vi "topicRequest_Reply_Decode.vi"(1 "Topic Request Reply":string) -> (0 "Topic Request Reply":T1)   [LabVIEW 2013]
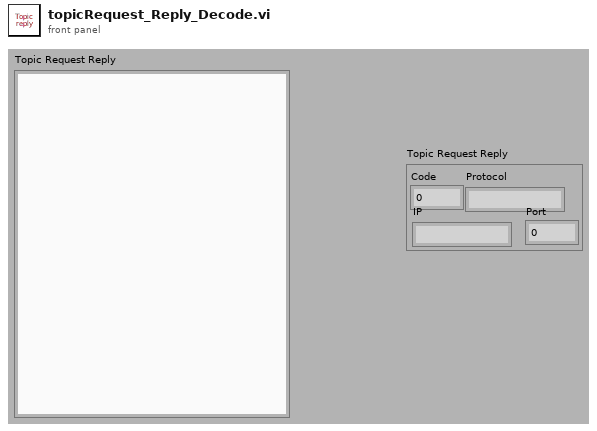
[diagram p1: front panel]
types:
  T1 = cluster{"Protocol":string, "Code":i32, "IP":string, "Port":i32}
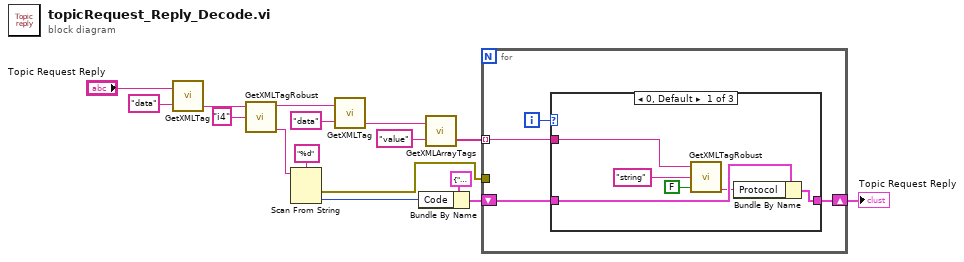
[diagram p0: block diagram]
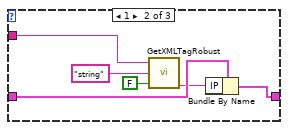
[diagram p2: hidden frame]
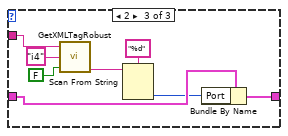
[diagram p3: hidden frame]
diagram:
  n1 = call "GetXMLTag.vi"("Tag"="data" ("ArrayTag"), "String"="Topic Request Reply") -> ("Value"=w12:string)  [unwired: 2 out]
  n2 = call "GetXMLTagRobust.vi"("Tag"="i4", "String"=w12) -> ("value"=w10:string, "String w/o Tag"=w4:string)  [unwired: 1 in, 2 out]
  n3 = Scan From String(format string="%d", input string=w10) -> (error out=w1:errorcluster, output 1=w9:i32)  [unwired: 3 in, 2 out]
  n4 = call "GetXMLTag.vi"("Tag"="data", "String"=w4) -> ("Value"=w3:string)  [unwired: 2 out]
  n5 = Bundle By Name(cluster=T1 {"Protocol"="", "Code"=0, "IP"="", "Port"=0} ("Topic Request Reply"), "Code"=w9) -> (w7:T1)
  n6 = call "GetXMLArrayTags.vi"("ArrayTag"="value", "String"=w3) -> ("Array"=w6:string[])  [unwired: 1 out]
  n7 = for {
    shift-right: [w19] -> w16
    shift-left: w7 -> [w20]
    tunnel: w6 -> [w18] mode=indexing
    tunnel: w1 -> [_]
    i -> [w17]
    n8 = case shown="0, Default" w17 {
      tunnel: w18 -> [w26 w32 w40]
      tunnel: w20 -> [w23 w30 w38]
      tunnel: [w21 w28 w37] -> w19
      frame 0, Default {
        n9 = call "GetXMLTagRobust.vi"("Tag only? (T)"=FALSE ("Tag only?"), "Tag"="string", "String"=w26) -> ("value"=w22:string)  [unwired: 3 out]
        n10 = Bundle By Name(cluster=w23, "Protocol"=w22) -> (w21:T1)
      }
      frame 1 {
        n11 = call "GetXMLTagRobust.vi"("Tag only? (T)"=FALSE ("Tag only?"), "Tag"="string", "String"=w32) -> ("value"=w29:string)  [unwired: 3 out]
        n12 = Bundle By Name(cluster=w30, "IP"=w29) -> (w28:T1)
      }
      frame 2 {
        n13 = call "GetXMLTagRobust.vi"("Tag only? (T)"=FALSE ("Tag only?"), "Tag"="i4", "String"=w40) -> ("value"=w35:string)  [unwired: 3 out]
        n14 = Scan From String(format string="%d", input string=w35) -> (output 1=w33:i32)  [unwired: 3 in, 3 out]
        n15 = Bundle By Name(cluster=w38, "Port"=w33) -> (w37:T1)
      }
    }
  }
  "Topic Request Reply" <- w16
